vi "Prefiltro.vi"(6 "y_k-2":dbl, 7 "y_k-1":dbl, 8 "x_k-2":dbl) -> (5 "y_k":dbl)   [LabVIEW 2018]
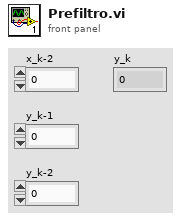
[diagram p1: front panel]
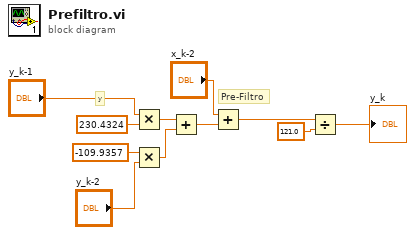
[diagram p0: block diagram]
diagram:
  # "Pre-Filtro"
  # "y"
  n1 = Multiply(x="y_k-1", y=230.4324) -> (x*y=w5:dbl)
  n2 = Multiply(x=-109.9357, y="y_k-2") -> (x*y=w6:dbl)
  n3 = Add(x=w5, y=w6) -> (x+y=w7:dbl)
  n4 = Add(x="x_k-2", y=w7) -> (x+y=w9:dbl)
  n5 = Divide(x=w9, y=121.0) -> (x/y=→"y_k":dbl)
